vi "Traverse-Move-Low.vi"(8 "error in":errorcluster, 9 "Trav Command":T1 items=["Read Position", "Move"], 10 "Settings":T3, 11 "Position Info IN":T2) -> (0 "error out":errorcluster, 3 "Position Info OUT":T2)   [LabVIEW 2017]
uses:
  TypeDefs/Position-Info-TD.ctl
  Settings/Settings-Control.ctl
  TypeDefs/Trav-Command-TD.ctl
  Settings/Traverse-Settings-Global.vi
panel:
  out "Speed Z":dbl
  out "Speed Y":dbl
  out "Speed X":dbl
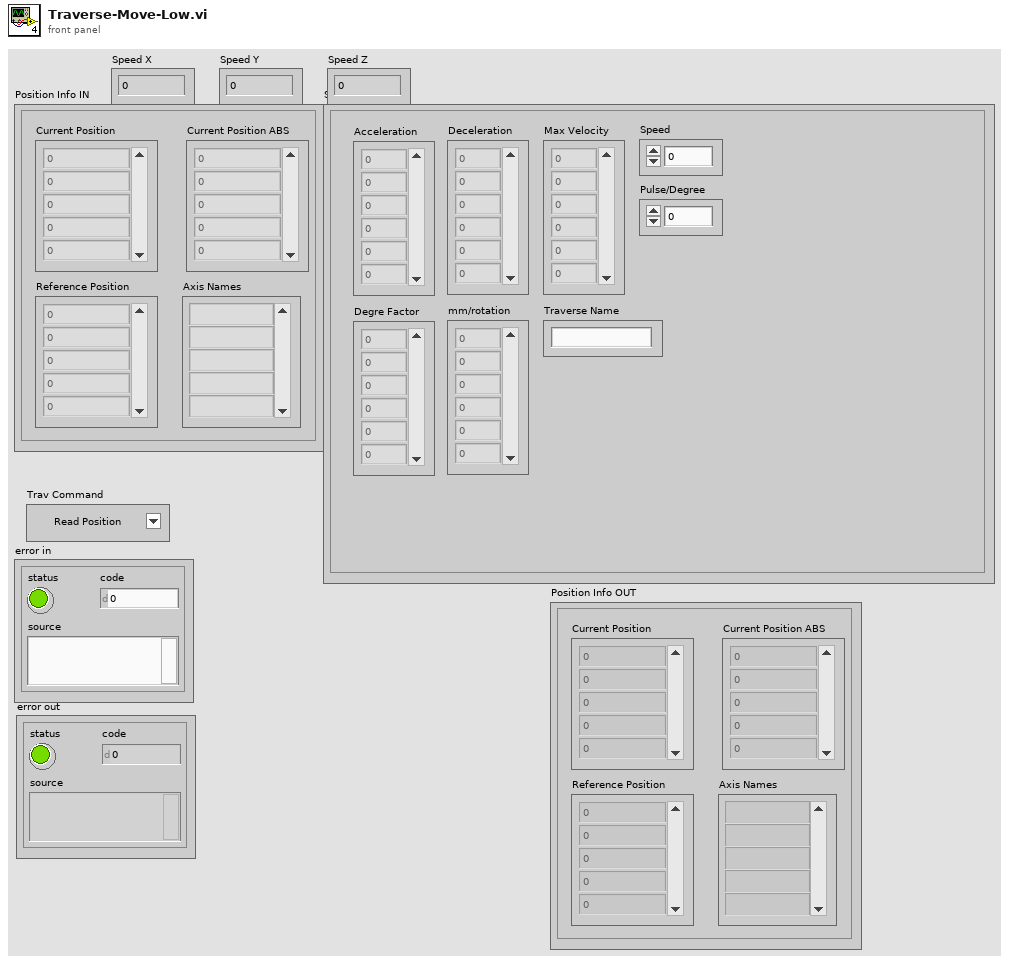
[diagram p1: front panel]
types:
  T1 = typedef "Trav-Command-TD.ctl" = u16
  T2 = typedef "Position-Info-TD.ctl" = cluster{"Current Position ABS":dbl[], "Current Position":dbl[], "Reference Position":dbl[], "Axis Names":string[]}
  T3 = typedef "Settings-Control.ctl" = cluster{"Acceleration":dbl[], "Deceleration":dbl[], "Max Velocity":dbl[], "Speed":dbl, "Pulse/Degree":dbl, "Degre Factor":dbl[], "mm/rotation":dbl[], "Traverse Name":string}
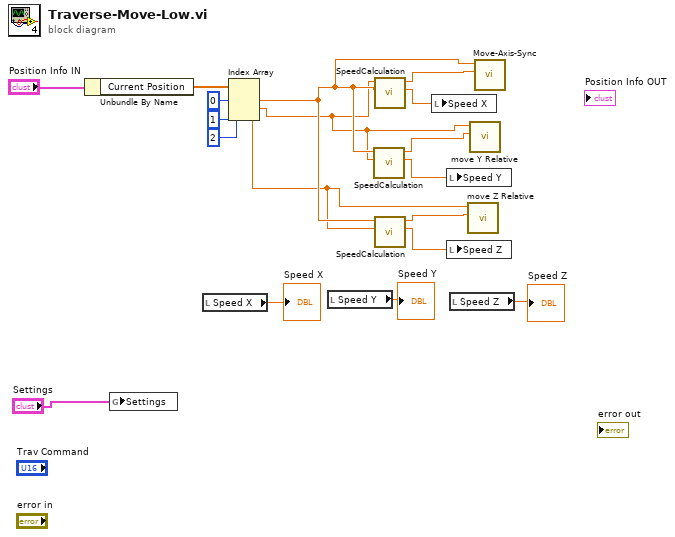
[diagram p0: block diagram]
diagram:
  n1 = Unbundle By Name("Position Info IN") -> ("Current Position"=w11:dbl[])
  n2 = global write "Traverse-Settings-Global.vi" "Settings"("Settings") -> ()
  n3 = local read "Speed X"() -> (→"Speed X":dbl)
  n4 = Index Array(array=w11, index #1=0 ("index"), index #2=1 ("index"), index #3=2 ("index")) -> (element #1=w10:dbl, element #2=w9:dbl, element #3=w8:dbl)
  n5 = local read "Speed Y"() -> (→"Speed Y":dbl)
  n6 = call "SpeedCalculation.vi"("Axis1"=w9, "Axis2"=w10) -> ("Speed mm/s"=w15:dbl, "Speed for card"=w17:dbl)  [unwired: 8 in]
  n7 = call "SpeedCalculation.vi"("Axis1"=w10, "Axis2"=w9) -> ("Speed mm/s"=w16:dbl, "Speed for card"=w13:dbl)  [unwired: 8 in]
  n8 = call "SpeedCalculation.vi"("Axis1"=w8, "Axis2"=w10) -> ("Speed mm/s"=w14:dbl, "Speed for card"=w18:dbl)  [unwired: 8 in]
  n9 = local write "Speed X"(w16) -> ()
  n10 = local write "Speed Y"(w15) -> ()
  n11 = local write "Speed Z"(w14) -> ()
  n12 = local read "Speed Z"() -> (→"Speed Z":dbl)
  n13 = call "move Z Relative.vi"("Z Speed"=w18, "z mm"=w8) -> ()  [unwired: 10 in]
  n14 = call "move Y Relative.vi"("Y Speed"=w17, "y mm"=w9) -> ()  [unwired: 10 in]
  n15 = call "Move-Axis-Sync.vi"("Speed X"=w13, "x mm"=w10) -> ()  [unwired: 10 in]
